vi "Fdx Get Rx Status.vi"(8 "error in":errorcluster, 11 "InstrumentHandle_port in":u32) -> (0 "error out":errorcluster, 1 "RxStatus":u32, 2 "Info":u32, 3 "InstrumentHandle_port out":u32)   [LabVIEW 2020, in "AIM664LV.lvlib"]
doc: "This function is used to retrieve the receiver status of the board."
uses:
  AIM664LV.lvlib
  AFDX_LibraryAdmin/FdxGlobalDllPath.vi
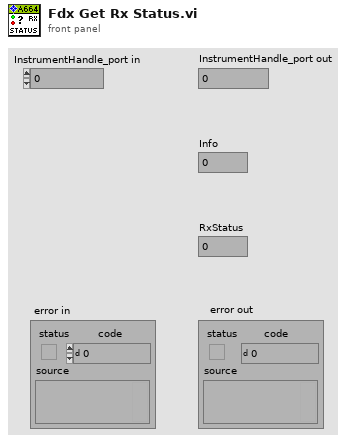
[diagram p1: front panel]
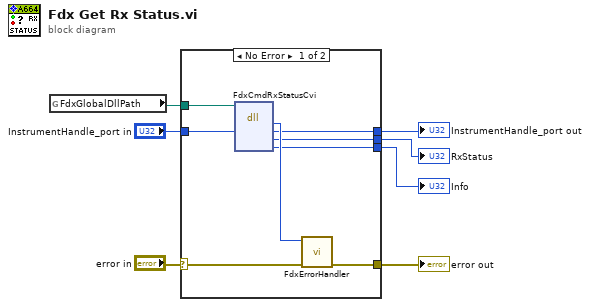
[diagram p0: block diagram]
diagram:
  n1 = global read "FdxGlobalDllPath.vi" "FdxGlobalDllPath"() -> (w5:path)
  n2 = case shown="No Error" "error in" {
    selector: "error in" -> [w14 w17]
    tunnel: [w15 w17] -> w7
    tunnel: w5 -> [w12 _]
    tunnel: "InstrumentHandle_port in" -> [w11 w16]
    tunnel: [w10 w16] -> w3
    tunnel: [w9 _] -> w2
    tunnel: [w8 _] -> w1
    frame No Error {
      n3 = dll-call lib="aim_fdx.19.dll" fn="FdxCmdRxStatusCvi"(path in=w12, "InstrumentHandle"=w11) -> ("status"=w13:i32, "InstrumentHandle"=w10:u32, "RxStatus"=w8:u32, "Info"=w9:u32)  [unwired: 2 in, 4 out]
      n4 = call "FdxErrorHandler.vi"("error in"=w14, "AIM Error"=w13) -> ("error out"=w15:errorcluster)  [unwired: 9 in]
    }
    frame Error {
    }
  }
  "error out" <- w7
  "InstrumentHandle_port out" <- w3
  "RxStatus" <- w1
  "Info" <- w2
